vi "controller_PID_NI.vi"(8 "error in (no error)":errorcluster, 10 "Reference Array":cluster{"Time":dbl[], "Reference":dbl[]}, 11 "Dynamic-System in":refnum<class "Dynamic-System.lvclass">) -> (0 "error out":errorcluster, 2 "Waveform Chart":dbl(graph), 3 "Dynamic-System out":refnum<class "Dynamic-System.lvclass">)   [LabVIEW 2025, in "Dynamic-System.lvclass"]
uses:
  Dynamic-System.lvclass
  Dynamic-System.lvclass/Dynamic-System.ctl
  <vilib>/addons/control/pid/pid.llb/PID (DBL).vi
  <vilib>/addons/control/pid/NI_PID_pid.lvlib
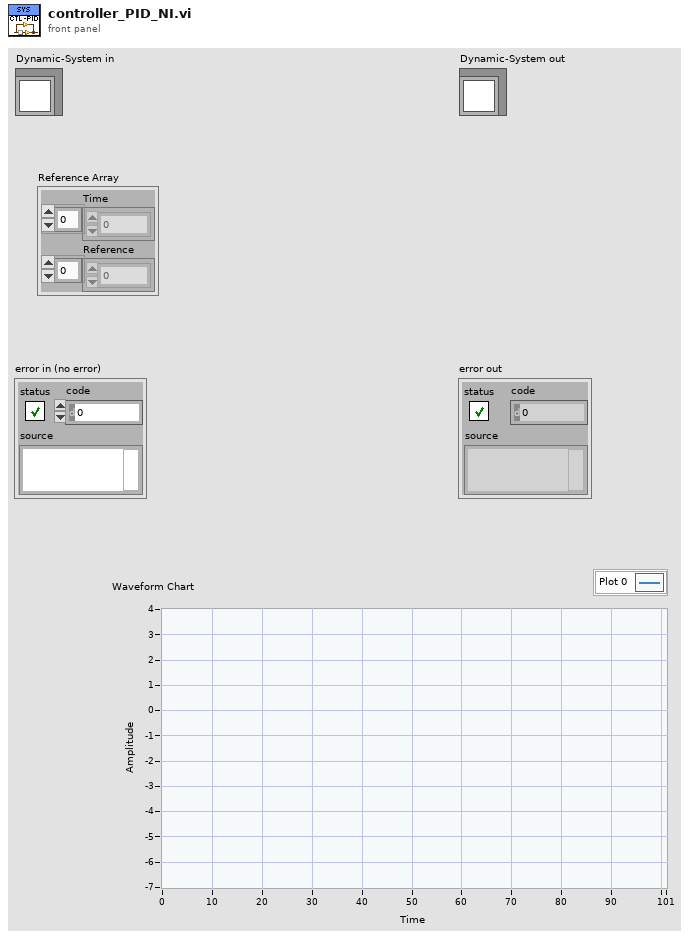
[diagram p1: front panel]
types:
  T1 = cluster{"proportional gain (Kc)":dbl, "integral time (Ti, min)":dbl, "derivative time (Td, min)":dbl}
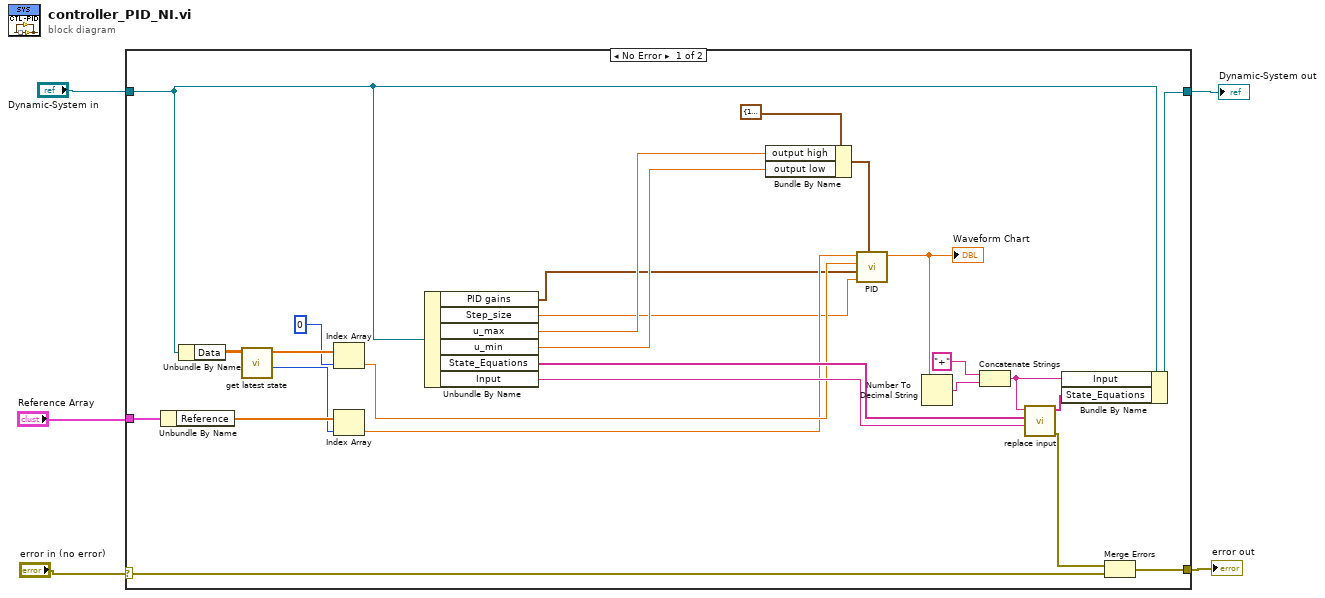
[diagram p0: block diagram]
diagram:
  n1 = case shown="No Error" "error in (no error)" {
    selector: "error in (no error)" -> [w17 w33]
    tunnel: [w15 w33] -> w3
    tunnel: [w22 w32] -> w4
    tunnel: "Dynamic-System in" -> [w25 w32]
    tunnel: "Reference Array" -> [w30 _]
    frame No Error {
      n2 = Unbundle By Name(w30) -> ("Reference"=w29:dbl[])
      n3 = Unbundle By Name(w25) -> ("Data"=w31:dbl[][])
      n4 = call "get latest state.vi"("t & X"=w31) -> ("end element"=w28:i32, "X_i"=w27:dbl[])  [unwired: 8 in, 1 out]
      n5 = Index Array(array=w27, index=0) -> (element=w10:dbl)
      n6 = Index Array(array=w29, index=w28) -> (element=w9:dbl)
      n7 = Unbundle By Name(w25) -> ("PID gains"=w6:T1, "Step_size"=w8:dbl, "u_max"=w12:dbl, "u_min"=w11:dbl, "State_Equations"=w19:string[], "Input"=w20:string)
      n8 = Bundle By Name(cluster=cluster{"output high":dbl, "output low":dbl} {"output high"=100.0, "output low"=-100.0} ("output range"), "output high"=w12, "output low"=w11) -> (w13:cluster{"output high":dbl, "output low":dbl})
      n9 = call-poly <vilib>:"PID.vi"("output range"=w13, "dt (s)"=w8, "PID gains"=w6, "process variable"=w10, "setpoint"=w9) -> ("output"=w7:dbl)  [unwired: 5 in, 1 out]
      "Waveform Chart" <- w7
      n10 = Number To Decimal String(number=w7) -> (decimal integer string=w24:string)  [unwired: 1 in]
      n11 = Concatenate Strings("+" ("string"), w24) -> (w21:string)
      n12 = call "replace input.vi"("Previous Input"=w20, "State_Equations in"=w19, "New Input"=w21) -> ("error out"=w16:errorcluster, "State_Equations out"=w18:string[])  [unwired: 7 in]
      n13 = Bundle By Name(cluster=w25, "Input"=w21, "State_Equations"=w18) -> (w22:refnum<class "Dynamic-System.lvclass">)
      n14 = Merge Errors(w16, w17) -> (w15:errorcluster)
    }
    frame Error {
    }
  }
  "error out" <- w3
  "Dynamic-System out" <- w4
